vi "XYZ Stage Driver (ver 2).vi"(11 "UI elements cluster":T1) -> (0 "error out (no error)":errorcluster)   [LabVIEW 2020]
uses:
  Typedefs/XYZ stage states.ctl
  Typedefs/UI ctrl refs cluster.ctl
  Typedefs/Laser control knob.ctl
  Typedefs/Frame Size.ctl
  Typedefs/Plane Mode.ctl
  Typedefs/PMT control knob.ctl
  Typedefs/XY Stage_Move.ctl
  Typedefs/test_fpga_control.ctl
  Acquisition/Typedefs/Ref DAQ Param.ctl
  User Interface/Misc/Experiment Type.ctl
  User Interface/Misc/Biology Information.ctl
  typedefs/XYZControlConfig.ctl
  Globals/gl_XYZStage globals.vi
  Global Variables/General Globals.vi
  Global Variables/gl_UI Ctrl Refs.vi
panel:
  in  "error in (no error)":errorcluster
  out "Interrupt loop itr":i32
  out "XYZ stage initialised":bool
  out "Motor driver loop itr":i32
  out "Command":T2
  out "Coordinates":cluster{"X":sgl, "Y":sgl, "Z":sgl}
  out "internal error cluster":errorcluster
  # "XYZ STAGE DRIVER"
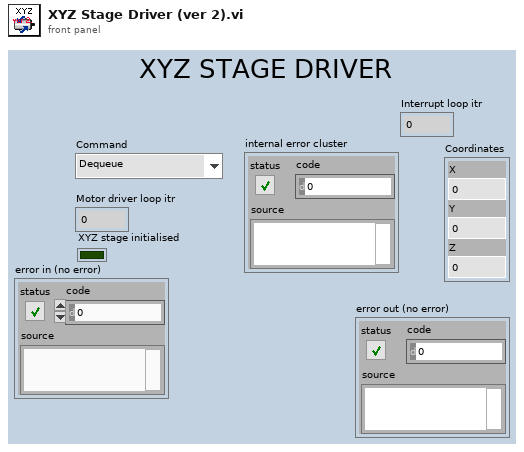
[diagram p1: front panel]
types:
  T1 = typedef "UI ctrl refs cluster.ctl" = cluster{"Top level VI path":path, "Top level VI ref":refnum<vi>, "User menu ref":refnum<k9>, "Sub Panel control":refnum<vi>, "Imaging Param Tab":refnum<vi>, "Occurrence-Start drivers":refnum<k4>, "Occurrence-Speed logging initialised":refnum<k4>, "Occurrence-XYZ stage initialised":refnum<k4>, "Exit button":refnum<vi>, "Status ind":refnum<vi>, "Set as origin":refnum<vi>, "Speed Logging":refnum<vi>, "Time Lapse":refnum<vi>, "Live Imaging":refnum<vi>, "AOL Z Stack":refnum<vi>, "Motor Z Stack":refnum<vi>, "Funct Acq button":refnum<vi>, "Hard Shutter":refnum<vi>, "Virtual Shutter":refnum<vi>, "Laser Power":refnum<vi>, "AOL Mode":refnum<vi>, "Frame Size":refnum<vi>, "Field of View":refnum<vi>, "Dwell Time":refnum<vi>, "Zoom":refnum<vi>, "AOL Z":refnum<vi>, "Objective":refnum<vi>, "Axis":refnum<vi>, "Paths & Names":refnum<vi>, "Experiment folder path (ind.)":refnum<vi>, "Last State (Ind.)":refnum<vi>, "Averages":refnum<vi>, "Angle (degrees)":refnum<vi>, "X centre":refnum<vi>, "Y centre":refnum<vi>, "Plane Mode":refnum<vi>, "# Planes":refnum<vi>, "Z Start":refnum<vi>, "Z Stop":refnum<vi>, "Z Step":refnum<vi>, "PMT 1":refnum<vi>, "PMT 2":refnum<vi>, "Stage XYZ Position":refnum<vi>, "Pockels@Z Start":refnum<vi>, "Pockels@Z Stop":refnum<vi>, "Obtain Z Start":refnum<vi>, "Obtain Z Stop":refnum<vi>, "Live stim.trig.period":refnum<vi>, "Live stim.trig.enable":refnum<vi>, "Movement Correction":refnum<vi>, "Load Reference Image":refnum<vi>, "XY Stage Move":refnum<vi>, "MovCor Cluster":refnum<vi>, "RefDAQParam":refnum<vi>, "Funct. Acq. Pockels Modulation":refnum<vi>, "Ref Laser Power":refnum<vi>, "Enable Video Recording":refnum<vi>, "Video Record-Live Imaging":refnum<vi>, "Video Record-Funct acq":refnum<vi>, "Reference Source":refnum<vi>, "AOL Z-stack Chirps Ready (ind)":refnum<vi>, "Target time between mov.cor. ref triggers (ms)":refnum<vi>, "Funct. Acq. Ref frame save":refnum<vi>, "Tracking button":refnum<vi>, "Show ref plots window":refnum<vi>, "Center freq ind (nm)":refnum<vi>, "Pickup mode (ind)":refnum<vi>, "Logging queue (ind)":refnum<vi>, "Back aperture power (ind.)":refnum<vi>, "Power after objective (ind.)":refnum<vi>, "Switch user":refnum<vi>, "Ls1 Conn. Status":refnum<vi>, "Ls1Tuning Status":refnum<vi>, "Ls1 Faults":refnum<vi>, "Ls1 Connection":refnum<vi>, "Ls1 Mode":refnum<vi>, "Ls1 POWER [mW]":refnum<vi>, "Ls1Shutter":refnum<vi>, "Ls1 Wavelength":refnum<vi>, "Ls1 Note":refnum<vi>, "Ls1 Confirm Wav":refnum<vi>, "Ls1 PreChrp Prism1":refnum<vi>, "Ls1 PreChrp Prism2":refnum<vi>, "Ls1 wav top Ind":refnum<vi>, "Ls1 power top Ind":refnum<vi>, "Ls1 Pump peak Hold":refnum<vi>, "Ls1 Status Ind":refnum<vi>, "Ls1 wav cancel":refnum<vi>, "Experiment Type":refnum<vi>, "Biology Information":refnum<vi>, "Camera recording status":refnum<vi>, "Optimise Obj. Pos.":refnum<vi>}
  T2 = typedef "XYZ stage states.ctl" = enum16{"Dequeue", "Initialize", "Read Position", "Read Speed Setting", "Move", "Set Max Speed", "Reset Axis", "Stop all movement"}
  T3 = typedef "XYZControlConfig.ctl" = enum16{"None", "XYZ", "XY-Z", "X-Y-Z", "Z"}
  T4 = typedef "TranslationStageControlInfo.ctl" = cluster{"CommsProtocol.lvclass":refnum<class "CommsProtocol.lvclass">, "CommsProtocol.lvclass 2":refnum<class "CommsProtocol.lvclass">, "CommsProtocol.lvclass 3":refnum<class "CommsProtocol.lvclass">, "XYZ Control Config":T3, "Translation Stage Description":string}
  T5 = typedef "XYZ stage data.ctl" = cluster{"Command":T2, "Channel":T6, "X":sgl, "Y":sgl, "Z":sgl, "Speed":i32, "Zero":bool, "Use acknowledgement?":bool}
  T6 = typedef "XYZ channel ring.ctl" = string
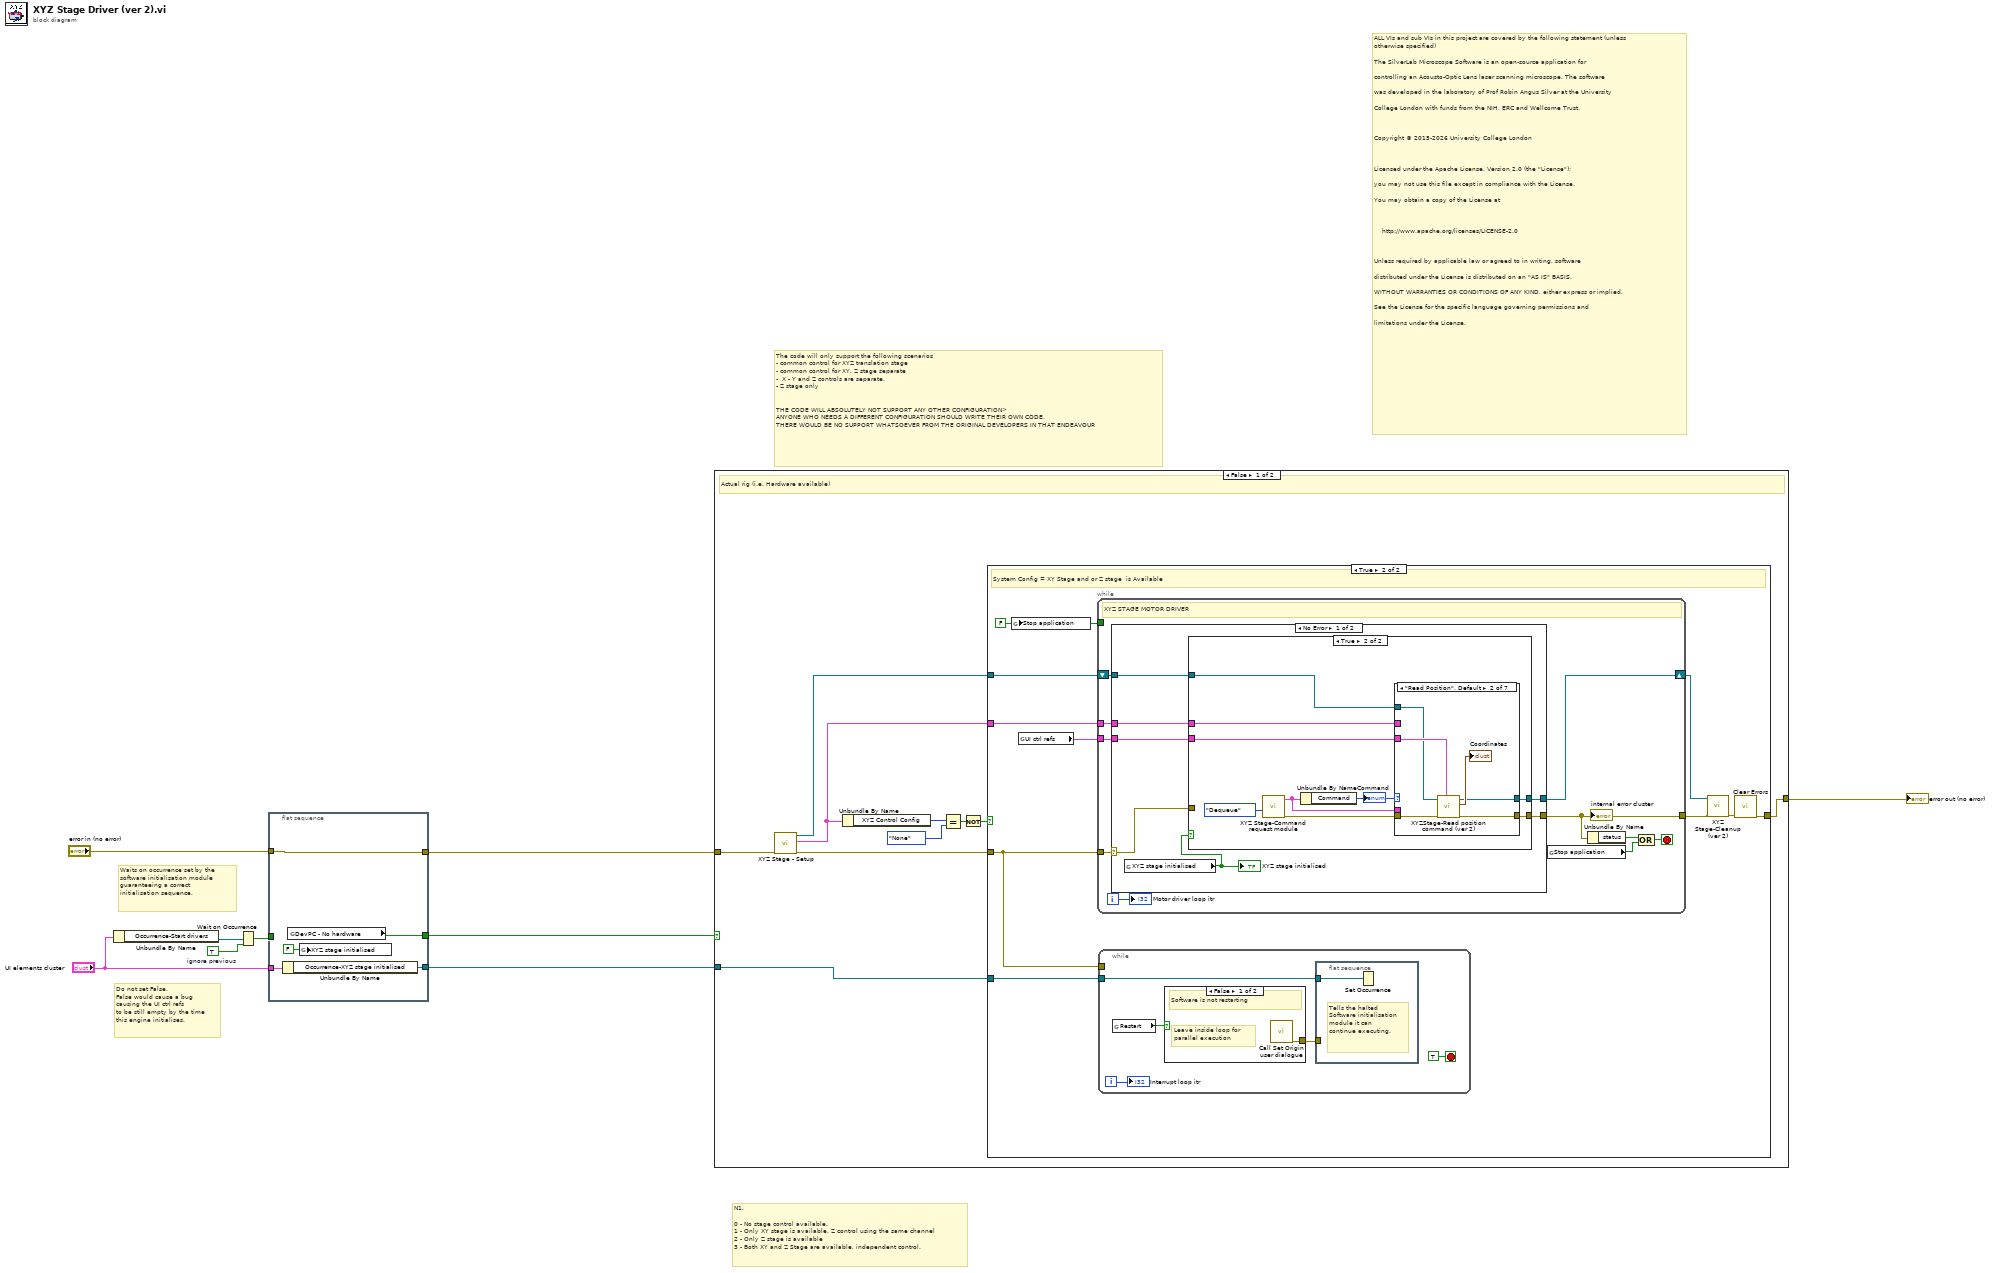
[diagram p0: block diagram]
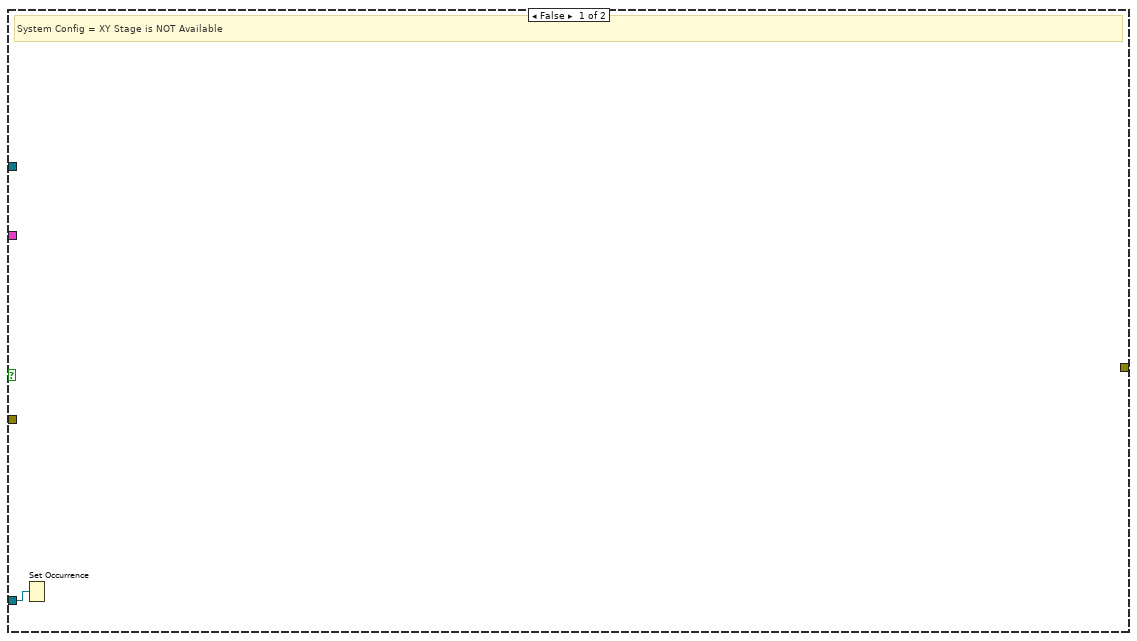
[diagram p2: hidden frame]
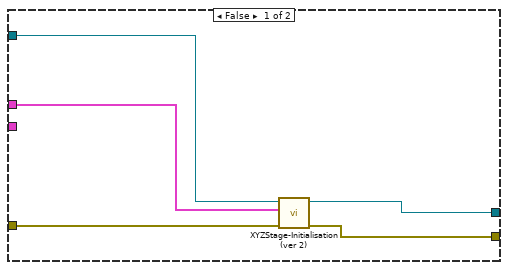
[diagram p4: hidden frame]
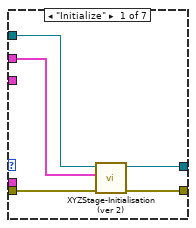
[diagram p5: hidden frame]
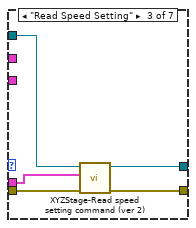
[diagram p6: hidden frame]
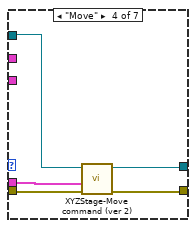
[diagram p7: hidden frame]
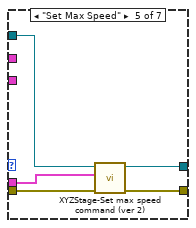
[diagram p8: hidden frame]
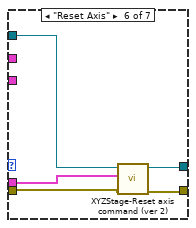
[diagram p9: hidden frame]
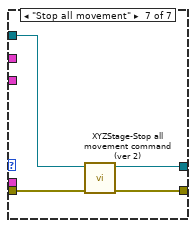
[diagram p10: hidden frame]
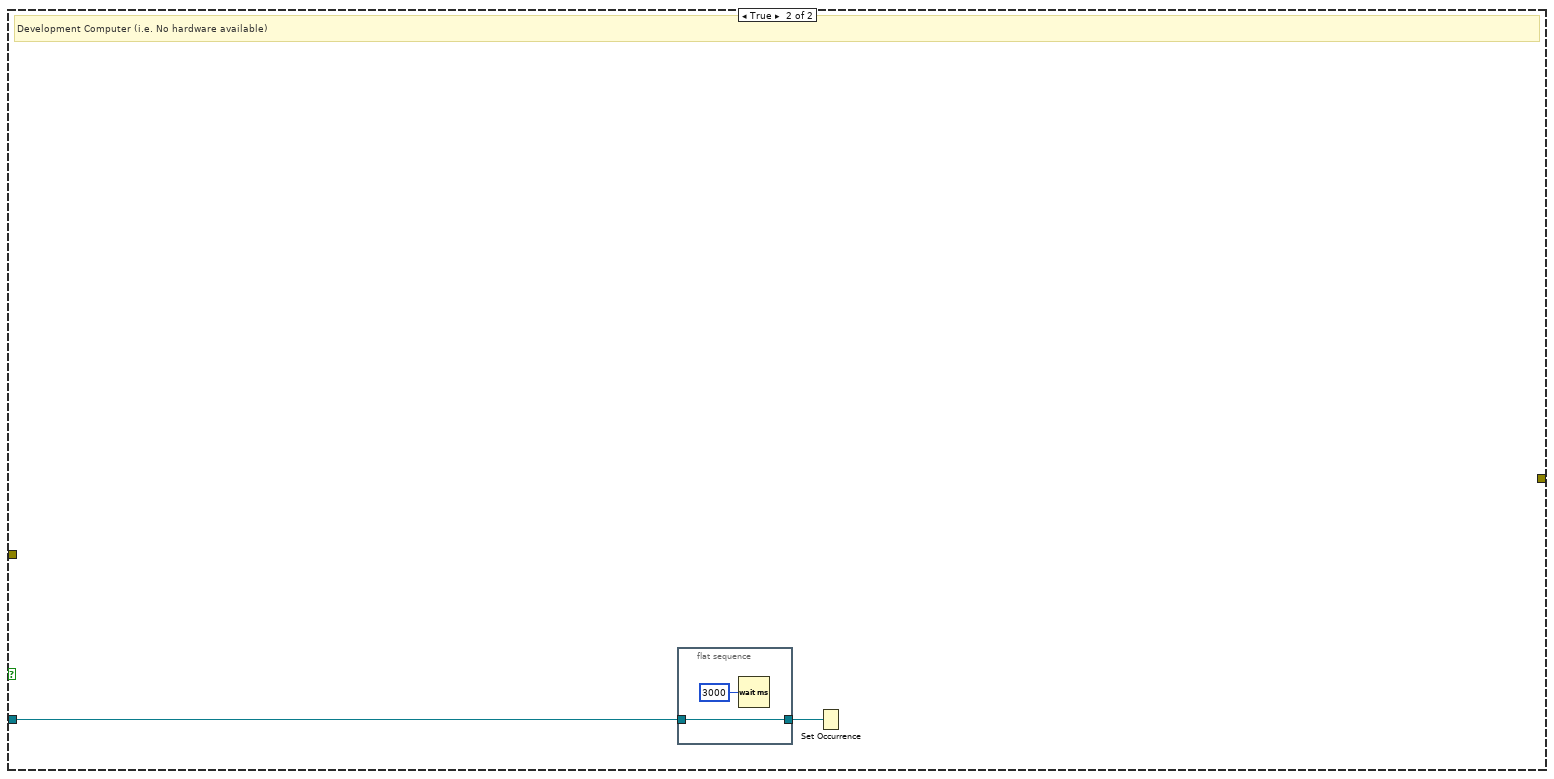
[diagram p12: hidden frame]
diagram:
  w5 = TRUE  # ignore previous
  # "ALL VIs and sub VIs in this project are covered by the following statement (unless \notherwise specified)\n\nThe SilverLab Microscope Software is an open-source application for\n\ncontrolling an Acousto-Optic Lens laser scanning microscope. The software\n\nwas developed in the laboratory of Prof Robin Angus Silver at the University\n\nCollege London with funds from the NIH, ERC and Wellcome Trust.\n\n \n\nCopyright © 2015-2026 University College London\n\n \n\nLicensed under the Apache License, Version 2.0 (the \"License\");\n\nyou may not use this file except in compliance with the License.\n\nYou may obtain a copy of the License at\n\n \n\n    http://www.apache.org/licenses/LICENSE-2.0\n\n \n\nUnless required by applicable law or agreed to in writing, software\n\ndistributed under the License is distributed on an \"AS IS\" BASIS,\n\nWITHOUT WARRANTIES OR CONDITIONS OF ANY KIND, either express or implied.\n\nSee the License for the specific language governing permissions and\n\nlimitations under the License."
  # "The code will only support the following scenarios\n- common control for XYZ translation stage\n- common control for XY, Z stage separate\n-  X - Y and Z controls are separate.\n- Z stage only\n\n\nTHE CODE WILL ABSOLUTELY NOT SUPPORT ANY OTHER CONFIGURATION>\nANYONE WHO NEEDS A DIFFERENT CONFIGURATION SHOULD WRITE THEIR OWN CODE. \nTHERE WOULD BE NO SUPPORT WHATSOEVER FROM THE ORIGINAL DEVELOPERS IN THAT ENDEAVOUR"
  # "N1. \n\n0 - No stage control available.\n1 - Only XY stage is available. Z control using the same channel\n2 - Only Z stage is available\n3 - Both XY and Z Stage are available, independent control."
  # "Do not set False.\nFalse would cause a bug\ncausing the UI ctrl refs\nto be still empty by the time\nthis engine initialises."
  # "Waits on occurrence set by the software initialisation module guaranteeing a correct initialisation sequence."
  n1 = Unbundle By Name("UI elements cluster") -> ("Occurrence-Start drivers"=w4:refnum<k4>)
  n2 = Wait on Occurrence(1:w5, 2:w4) -> (0:w6:bool)  [unwired: 1 in]
  n3 = flat-sequence {
    tunnel: [w14] -> w3
    tunnel: "UI elements cluster" -> [w13]
    tunnel: [w12] -> w8
    tunnel: w6 -> [_]
    tunnel: [w10] -> w2
    tunnel: "error in (no error)" -> [w10]
    frame #0 {
      n4 = Unbundle By Name(w13) -> ("Occurrence-XYZ stage initialised"=w12:refnum<k4>)
      n5 = global read "General Globals.vi" "DevPC - No hardware"() -> (w14:bool)
      n6 = global write "gl_XYZStage globals.vi" "XYZ stage initialised"(FALSE ("XYZ stage initialised")) -> ()
    }
  }
  n7 = case shown="False" w3 {
    tunnel: [w24 _] -> w9
    tunnel: w8 -> [w23 w112]
    tunnel: w2 -> [w22 _]
    frame False {
      # "Actual rig (i.e. Hardware available)"
      n8 = call "XYZ Stage - Setup.vi"("error in (no error)"=w22) -> ("error out"=w17:errorcluster, "Stage Comms"=w16:T4, "XYZ Stage Control.lvclass"=w15:refnum<class "XYZ Stage Control.lvclass">)  [unwired: 8 in]
      n9 = Unbundle By Name(w16) -> ("XYZ Control Config"=w21:T3)
      n10 = Equal?(x=w21, y=XYZControlConfig."None") -> (x = y?=w19:bool)
      n11 = Not(x=w19) -> (.not. x?=w18:bool)
      n12 = case shown="True" w18 {
        tunnel: w23 -> [w25 w35]
        tunnel: w17 -> [_ w33]
        tunnel: [_ w32] -> w24
        tunnel: w15 -> [_ w30]
        tunnel: w16 -> [_ w29]
        frame False {
          # "System Config = XY Stage is NOT Available"
          n13 = Set Occurrence(w25) -> ()
        }
        frame True {
          w34 = FALSE ("Stop application")
          # "System Config = XY Stage and or Z stage  is Available"
          n14 = global write "General Globals.vi" "Stop application"(w34) -> ()
          n15 = global read "gl_UI Ctrl Refs.vi" "UI ctrl refs"() -> (w31:T1)
          n16 = while {
            tunnel: w33 -> [w50]
            tunnel: [w48] -> w28
            tunnel: w34 -> [_]
            tunnel: w31 -> [w47]
            shift-right: [w44] -> w27
            shift-left: w30 -> [w45]
            tunnel: w29 -> [w43]
            i -> [w46]
            stop <- w52 stop-if-true
            # "XYZ STAGE MOTOR DRIVER"
            n17 = case shown="No Error" w50 {
              selector: w50 -> [w53 w110]
              tunnel: [w59 w110] -> w48
              tunnel: w47 -> [w57 _]
              tunnel: w45 -> [w56 w109]
              tunnel: [w55 w109] -> w44
              tunnel: w43 -> [w54 _]
              frame No Error {
                n18 = global read "gl_XYZStage globals.vi" "XYZ stage initialised"() -> (w58:bool)
                "XYZ stage initialised" <- w58
                n19 = case shown="True" w58 {
                  tunnel: [w64 w73] -> w59
                  tunnel: w57 -> [_ w68]
                  tunnel: w56 -> [w62 w67]
                  tunnel: [w63 w66] -> w55
                  tunnel: w54 -> [w61 w65]
                  tunnel: w53 -> [w60 _]
                  frame False {
                    n20 = call "XYZStage-Initialisation (ver 2).vi"("Error In"=w60, "Stage Comms"=w61, "XYZ Stage Control.lvclass"=w62) -> ("Error Out"=w64:errorcluster, "XYZ Stage Control out"=w63:refnum<class "XYZ Stage Control.lvclass">)  [unwired: 7 in]
                  }
                  frame True {
                    n21 = call "XYZ Stage-Command request module.vi"("Command"=XYZ_stage_states."Dequeue") -> ("error out"=w71:errorcluster, "XYZ Stage dequeued data"=w70:T5)  [unwired: 6 in, 3 out]
                    n22 = Unbundle By Name(w70) -> ("Command"=w72:T2)
                    "Command" <- w72
                    n23 = case shown="\"Read Position\", Default" w72 {
                      tunnel: w70 -> [_ _ w85 w90 w97 w100 _]
                      tunnel: w71 -> [w78 w84 w89 w94 w99 w104 w108]
                      tunnel: [w77 w83 w88 w93 w98 w103 w107] -> w73
                      tunnel: w68 -> [_ w81 _ _ _ _ _]
                      tunnel: w67 -> [w74 w80 w87 w91 w96 w102 w106]
                      tunnel: [w76 w79 w86 w92 w95 w101 w105] -> w66
                      tunnel: w65 -> [w75 _ _ _ _ _ _]
                      frame "Initialize" {
                        n24 = call "XYZStage-Initialisation (ver 2).vi"("Error In"=w78, "Stage Comms"=w75, "XYZ Stage Control.lvclass"=w74) -> ("Error Out"=w77:errorcluster, "XYZ Stage Control out"=w76:refnum<class "XYZ Stage Control.lvclass">)  [unwired: 7 in]
                      }
                      frame "Read Position", Default {
                        n25 = call "XYZStage-Read position command (ver 2).vi"("UI ctrl refs"=w81, "error in (no error)"=w84, "XYZ Stage Control.lvclass"=w80) -> ("error out"=w83:errorcluster, "Coordinates"=→"Coordinates":cluster{"X":sgl, "Y":sgl, "Z":sgl}, "XYZ Stage Control.lvclass"=w79:refnum<class "XYZ Stage Control.lvclass">)  [unwired: 6 in]
                      }
                      frame "Read Speed Setting" {
                        n26 = call "XYZStage-Read speed setting command (ver 2).vi"("error in (no error)"=w89, "XYZ Stage data to queue"=w85, "XYZ Stage Control.lvclass"=w87) -> ("error out"=w88:errorcluster, "XYZ Stage Control.lvclass"=w86:refnum<class "XYZ Stage Control.lvclass">)  [unwired: 7 in]
                      }
                      frame "Move" {
                        n27 = call "XYZStage-Move command (ver 2).vi"("Error In"=w94, "XYZ Stage data"=w90, "XYZ Stage Control in"=w91) -> ("Error Out"=w93:errorcluster, "XYZ Stage Control out"=w92:refnum<class "XYZ Stage Control.lvclass">)  [unwired: 6 in, 1 out]
                      }
                      frame "Set Max Speed" {
                        n28 = call "XYZStage-Set max speed command (ver 2).vi"("Error In"=w99, "XYZ Stage data"=w97, "XYZ Stage Control in"=w96) -> ("Error Out"=w98:errorcluster, "XYZ Stage Control out"=w95:refnum<class "XYZ Stage Control.lvclass">)  [unwired: 7 in]
                      }
                      frame "Reset Axis" {
                        n29 = call "XYZStage-Reset axis command (ver 2).vi"("error in (no error)"=w104, "XYZ Stage dequeued data"=w100, "XYZ Stage Control in"=w102) -> ("error out"=w103:errorcluster, "XYZ Stage Control out"=w101:refnum<class "XYZ Stage Control.lvclass">)  [unwired: 7 in]
                      }
                      frame "Stop all movement" {
                        n30 = call "XYZStage-Stop all movement command (ver 2).vi"("Error In"=w108, "XYZ Stage Control in"=w106) -> ("Error Out"=w107:errorcluster, "XYZ Stage Control out"=w105:refnum<class "XYZ Stage Control.lvclass">)  [unwired: 8 in]
                      }
                    }
                  }
                }
              }
              frame Error {
              }
            }
            "internal error cluster" <- w48
            n31 = global read "General Globals.vi" "Stop application"() -> (w49:bool)
            n32 = Unbundle By Name(w48) -> ("status"=w51:bool)
            n33 = Compound Arithmetic op=OR(w51, w49) -> (w52:bool)
            "Motor driver loop itr" <- w46
          }
          n34 = while {
            tunnel: w33 -> [_]
            tunnel: w35 -> [w38]
            i -> [w36]
            stop <- TRUE stop-if-true
            n35 = global read "General Globals.vi" "Restart"() -> (w37:bool)
            n36 = case shown="False" w37 {
              tunnel: [w41 _] -> w39
              frame False {
                # "Leave inside loop for parallel execution"
                # "Software is not restarting"
                n37 = call "Call Set Origin user dialogue.vi"() -> ("error out"=w41:errorcluster)  [unwired: 11 in]
              }
              frame True {
                # "Software Restarting"
              }
            }
            n38 = flat-sequence {
              tunnel: w39 -> [_]
              tunnel: w38 -> [w42]
              frame #0 {
                # "Tells the halted Software initialisation\nmodule it can continue executing."
                n39 = Set Occurrence(w42) -> ()
              }
            }
            "Interrupt loop itr" <- w36
          }
          n40 = call "XYZ Stage-Cleanup (ver 2).vi"("error in (no error)"=w28, "XYZ Stage Control in"=w27) -> ("error out"=w26:errorcluster)  [unwired: 8 in, 1 out]
          n41 = call <vilib>:"Clear Errors.vi"("error in (no error)"=w26) -> ("error out"=w32:errorcluster)  [unwired: 5 in, 1 out]
        }
      }
    }
    frame True {
      # "Development Computer (i.e. No hardware available)"
      n42 = flat-sequence {
        tunnel: w112 -> [w114]
        tunnel: [w114] -> w111
        frame #0 {
          n43 = Wait (ms)(milliseconds to wait=u32 3000) -> ()  [unwired: 1 out]
        }
      }
      n44 = Set Occurrence(w111) -> ()
    }
  }
  "error out (no error)" <- w9
